vi "Save Hidden Config.vi"(0 "EnumV":string, 1 "EnumRadio":string, 2 "DataFilePath":path, 7 "Profile":string[][](array[string]), 9 "Serial Numbers":string[](array[string]), 11 "Header Info":string[](array[string])) -> ()   [LabVIEW 2013]
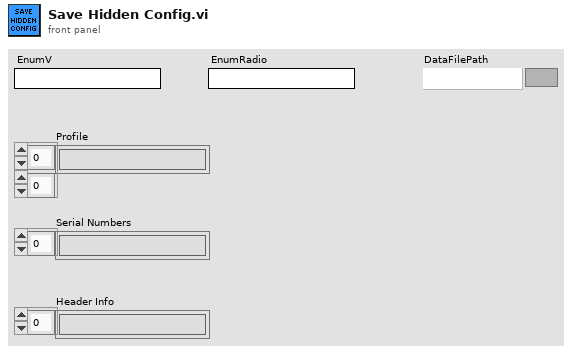
[diagram p1: front panel]
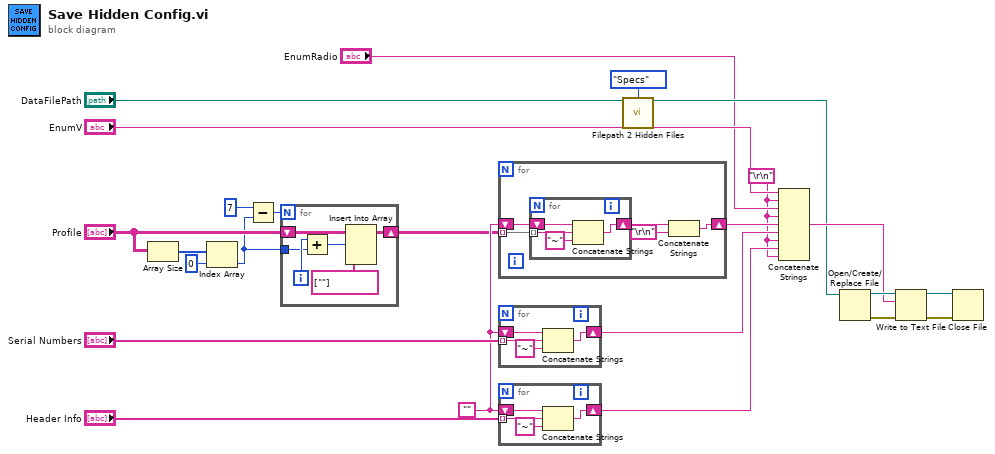
[diagram p0: block diagram]
diagram:
  w8 = ""
  w1 = "\r\n"
  n1 = Array Size(array="Profile") -> (size(s)=w24:i32[])
  n2 = Index Array(array=w24, index=0) -> (element=w4:i32)
  n3 = Subtract(x=7, y=w4) -> (x-y=w6:i32)
  n4 = for {
    N: w6 -> [_]
    shift-right: [w27] -> w3
    shift-left: "Profile" -> [w28]
    tunnel: w4 -> [w25]
    i -> [w26]
    n5 = Add(x=w26, y=w25) -> (x+y=w30:i32)
    n6 = Insert Into Array(array=w28, index (row)=w30, new element=string[] [""]) -> (w27:string[][])  [unwired: 1 in]
  }
  n7 = for {
    tunnel: w3 -> [w35] mode=indexing
    shift-right: [w32] -> w19
    shift-left: w8 -> [w34]
    n8 = for {
      tunnel: w35 -> [w39] mode=indexing
      shift-right: [w36] -> w33
      shift-left: w34 -> [w37]
      n9 = Concatenate Strings(w37, w39, "~" ("string")) -> (w36:string)
    }
    n10 = Concatenate Strings(w33, "\r\n") -> (w32:string)
  }
  n11 = for {
    tunnel: "Serial Numbers" -> [w43] mode=indexing
    shift-right: [w40] -> w18
    shift-left: w8 -> [w41]
    n12 = Concatenate Strings(w41, w43, "~" ("string")) -> (w40:string)
  }
  n13 = for {
    tunnel: "Header Info" -> [w47] mode=indexing
    shift-right: [w44] -> w17
    shift-left: w8 -> [w45]
    n14 = Concatenate Strings(w45, w47, "~" ("string")) -> (w44:string)
  }
  n15 = call "Filepath 2 Hidden Files.vi"("DataFilePath"="DataFilePath", "Enum"=enum16{"Data", "Stats", "Specs"}."Specs") -> ("HiddenFilePath"=w9:path)  [unwired: 13 in]
  n16 = Concatenate Strings("EnumV", w1, "EnumRadio", w1, w19, w18, w1, w17, w1) -> (w12:string)
  n17 = Open/Create/Replace File(file path (use dialog)=w9) -> (refnum out=w16:refnum<file>, error out=w14:errorcluster)  [unwired: 5 in, 1 out]
  n18 = Write to Text File(file (use dialog)=w16, text=w12, error in=w14) -> (refnum out=w15:refnum<file>, error out=w13:errorcluster)  [unwired: 1 in, 1 out]
  n19 = Close File(refnum=w15, error in=w13) -> ()  [unwired: 2 out]
